vi "Set Nested Item Visibility.vi"(8 "error in (no error)":errorcluster, 10 "Visible?":bool, 11 "MenuButton in":refnum<class "MenuButton.lvclass">) -> (0 "error out":errorcluster, 3 "MenuButton out":refnum<class "MenuButton.lvclass">)   [LabVIEW 2017, in "MenuButtons.lvlib" / "MenuButton.lvclass"]
uses:
  MenuButton.lvclass
  MenuButton.lvclass/MenuButton.ctl
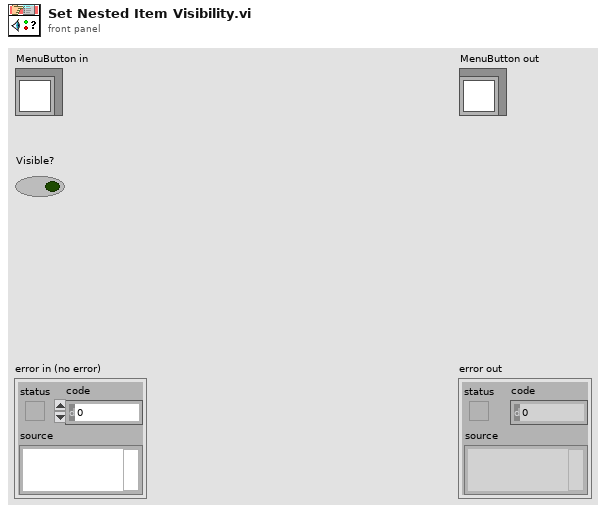
[diagram p1: front panel]
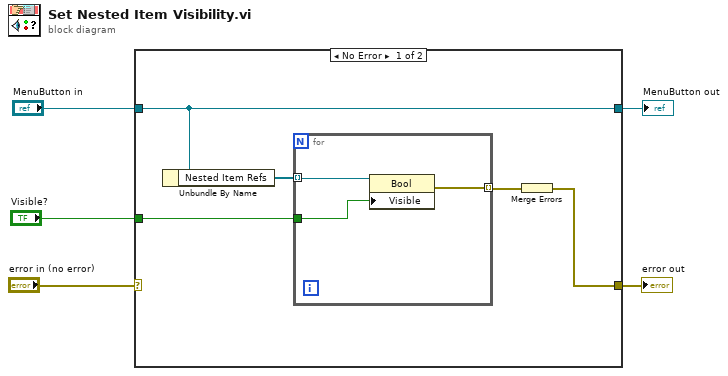
[diagram p0: block diagram]
diagram:
  n1 = case shown="No Error" "error in (no error)" {
    selector: "error in (no error)" -> [_ w15]
    tunnel: [w6 w15] -> w4
    tunnel: [w10 w14] -> w2
    tunnel: "MenuButton in" -> [w10 w14]
    tunnel: "Visible?" -> [w8 _]
    frame No Error {
      n2 = Unbundle By Name(w10) -> ("Nested Item Refs"=w9:refnum<vi>[])
      n3 = for {
        tunnel: w9 -> [w13] mode=indexing
        tunnel: w8 -> [w12]
        tunnel: [w11] -> w7 mode=indexing
        n4 = property class="Bool"(reference=w13, "Visible"=w12) -> (error out=w11:errorcluster)  [unwired: 1 in, 1 out]
      }
      n5 = Merge Errors(w7) -> (w6:errorcluster)
    }
    frame Error {
    }
  }
  "error out" <- w4
  "MenuButton out" <- w2
